vi "Tree Add Node.vi"(8 "error in (no error)":errorcluster, 9 "Usage":string, 10 "Name":string, 11 "Tree DVR in":refnum<data-value>) -> (0 "error out":errorcluster, 2 "Node out":refnum<data-value>, 3 "Tree DVR out":refnum<data-value>)   [LabVIEW 2012, in "MDSplus.lvlib"]
doc: "Add a new node to the tree open for edit."
uses:
  <vilib>/MDSplus/Library/MDSplus.lvlib
  <vilib>/MDSplus/Classes/Tree_Class/Tree.lvclass
  <vilib>/MDSplus/Classes/Data_Class/TreeNode_Class/TreeNode.lvclass
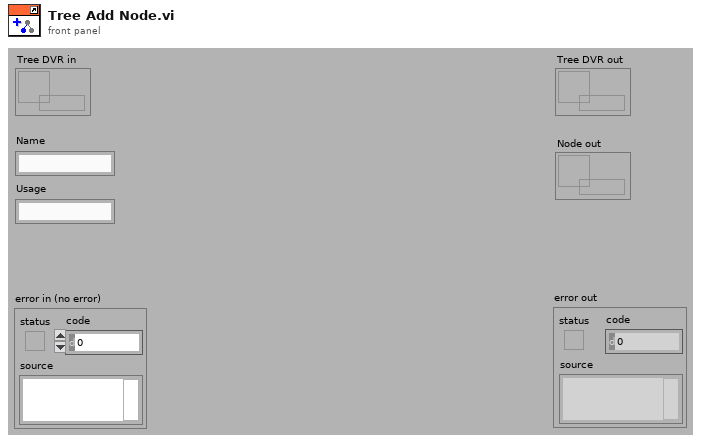
[diagram p1: front panel]
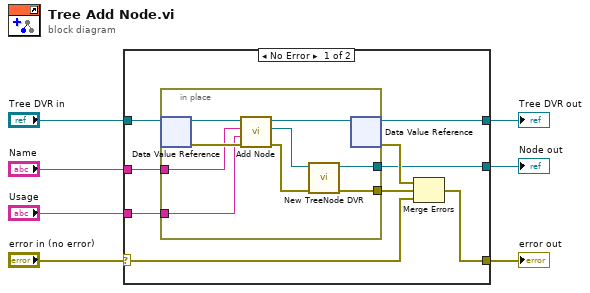
[diagram p0: block diagram]
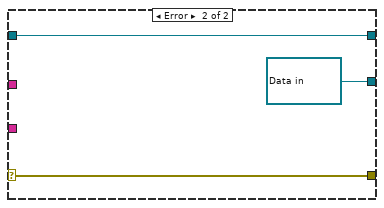
[diagram p2: hidden frame]
diagram:
  n1 = case shown="No Error" "error in (no error)" {
    selector: "error in (no error)" -> [w15 w28]
    tunnel: "Tree DVR in" -> [w16 w27]
    tunnel: [w13 w28] -> w7
    tunnel: [w12 w27] -> w4
    tunnel: [w8 refnum<data-value> refnum ("TreeNode DVR out")] -> w2
    tunnel: "Name" -> [w11 _]
    tunnel: "Usage" -> [w10 _]
    frame No Error {
      n2 = in-place {
        in-place-border: [w17] -> w9
        in-place-border: [w19] -> w8
        in-place-border: w11 -> [w22]
        in-place-border: w10 -> [w21]
        n3 = in-place-dvr #1(w16) -> (w25:refnum<class "Tree.lvclass">, w23:errorcluster)
        n4 = call-dynamic "Add Node.vi"("error in (no error)"=w23, "Usage"=w21, "Name"=w22, "Tree in"=w25) -> ("error out"=w18:errorcluster, "Node out"=w20:refnum<class "TreeNode.lvclass">, "Tree out"=w24:refnum<class "Tree.lvclass">)  [unwired: 5 in]
        n5 = call <vilib>:"New TreeNode DVR.vi"("error in (no error)"=w18, "TreeNode in"=w20) -> ("error out"=w17:errorcluster, "TreeNode DVR out"=w19:refnum<data-value>)  [unwired: 8 in]
        n6 = in-place-dvr #1(w24) -> (w12:refnum<data-value>, w14:errorcluster)
      }
      n7 = Merge Errors(w14, w9, w15) -> (w13:errorcluster)
    }
    frame Error {
    }
  }
  "error out" <- w7
  "Tree DVR out" <- w4
  "Node out" <- w2
